vi "Report init.vi"(9 "Baugruppe":string, 10 "Artikelnummer":string, 11 "Prüfer":string) -> (1 "Baugruppe (Ausgang)":string, 2 "obnr (Ausgang)":string, 3 "Prüfer (Ausgang)":string)   [LabVIEW 2013, in "DataCreation.lvlib"]
uses:
  lib/DataCreation.lvlib
panel:
  in  "OK-Schaltfläche":bool
  # "unterstützte EMV-Prüfberichterstellung"
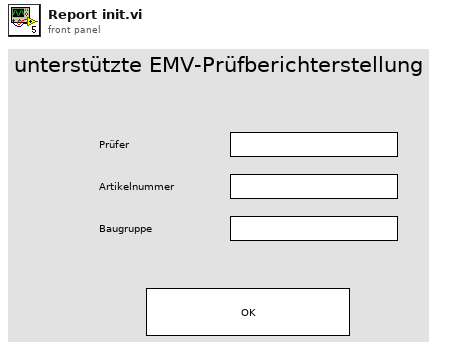
[diagram p1: front panel]
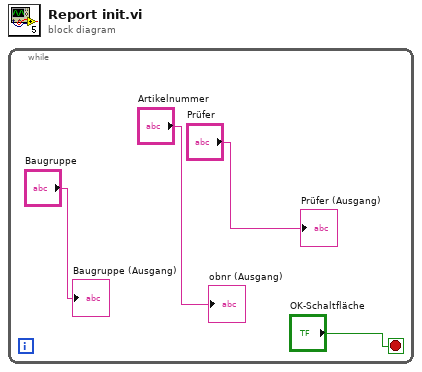
[diagram p0: block diagram]
diagram:
  n1 = while {
    stop <- "OK-Schaltfläche" stop-if-true
    "Baugruppe (Ausgang)" <- "Baugruppe"
    "Prüfer (Ausgang)" <- "Prüfer"
    "obnr (Ausgang)" <- "Artikelnummer"
  }
